vi "Check Wavename Length.vi"(2 "error in (no error)":errorcluster, 3 "Wavename":string) -> (0 "error out":errorcluster, 1 "Wavename out":string)   [LabVIEW 2019, in "Data.ITX.lvclass"]
uses:
  Data.ITX.lvclass
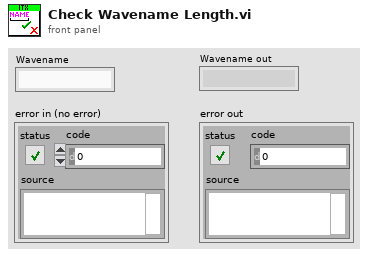
[diagram p1: front panel]
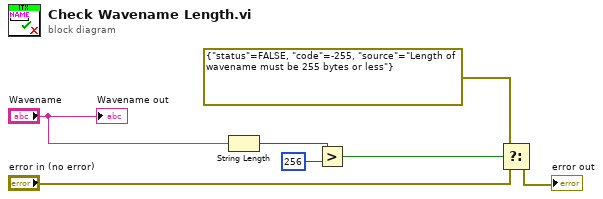
[diagram p0: block diagram]
diagram:
  n1 = String Length(string="Wavename") -> (length=w3:i32)
  n2 = Greater?(x=w3, y=256) -> (0:w5:bool)
  n3 = Select(t=errorcluster {"status"=FALSE, "code"=-255, "source"="Length of wavename must be 255 bytes or less"} ("error constant"), s=w5, f="error in (no error)") -> (s? t:f=→"error out":errorcluster)
  "Wavename out" <- "Wavename"
